vi "Up Down Counter.vi"() -> ()   [LabVIEW 2016]
panel:
  out "x":dbl
  out "x+y":dbl
  in  "Up or Down":bool
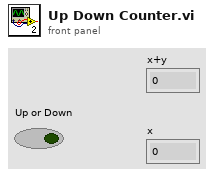
[diagram p1: front panel]
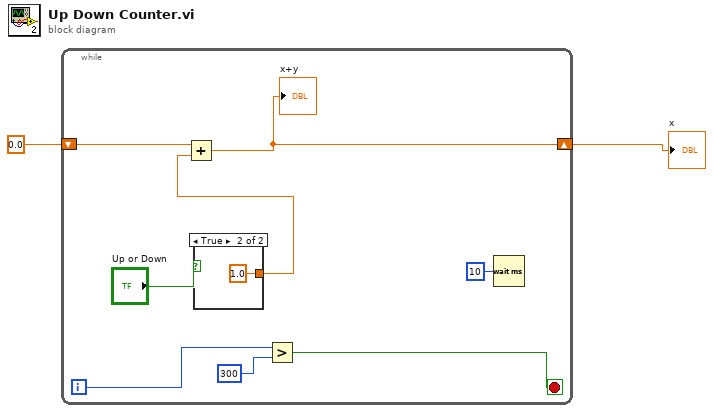
[diagram p0: block diagram]
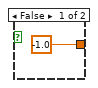
[diagram p2: hidden frame]
diagram:
  n1 = while {
    shift-right: [w8] -> w1
    shift-left: 0.0 ("x+y") -> [w9]
    i -> [w6]
    stop <- w4 stop-if-true
    n2 = case shown="True" "Up or Down" {
      tunnel: [-1.0 ("x") 1.0 ("x")] -> w7
      frame False {
      }
      frame True {
      }
    }
    n3 = Add(x=w9, y=w7) -> (x+y=w8:dbl)
    "x+y" <- w8
    n4 = Greater?(x=w6, y=300) -> (0:w4:bool)
    n5 = Wait (ms)(milliseconds to wait=u32 10) -> ()  [unwired: 1 out]
  }
  "x" <- w1
